vi "NumeroMisureRes.vi"() -> ()   [LabVIEW 2019]
panel:
  out "Numero misure resistomat":dbl
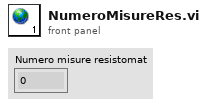
[diagram p1: front panel]
diagram:
